vi "ExecLog_AddLogEntry.vi"(2 "Msg":string, 4 "EnableListDisplay":bool, 5 "Reset":bool, 6 "ReadLog":bool, 7 "FileRef":refnum<file>, 8 "error in":errorcluster, 9 "Force":bool, 10 "Code":i16=-1, 11 "Enable":bool) -> (0 "Log":string[][](array[string]), 1 "NewMsg":bool, 3 "ErrorOut":errorcluster)   [LabVIEW 2017]
doc: "Adds a log entry.\nFilters out duplicate messages and includes only the first and last. Duplicates can be either identified by identical text or by the same error code.\nCode is only ignored if zero."
uses:
  ExecLog_Type.ctl
panel:
  in  "LogType":T1
  out "call chain 2":string[](array[string])
  in  "Multicolumn Listbox":i32(listbox)
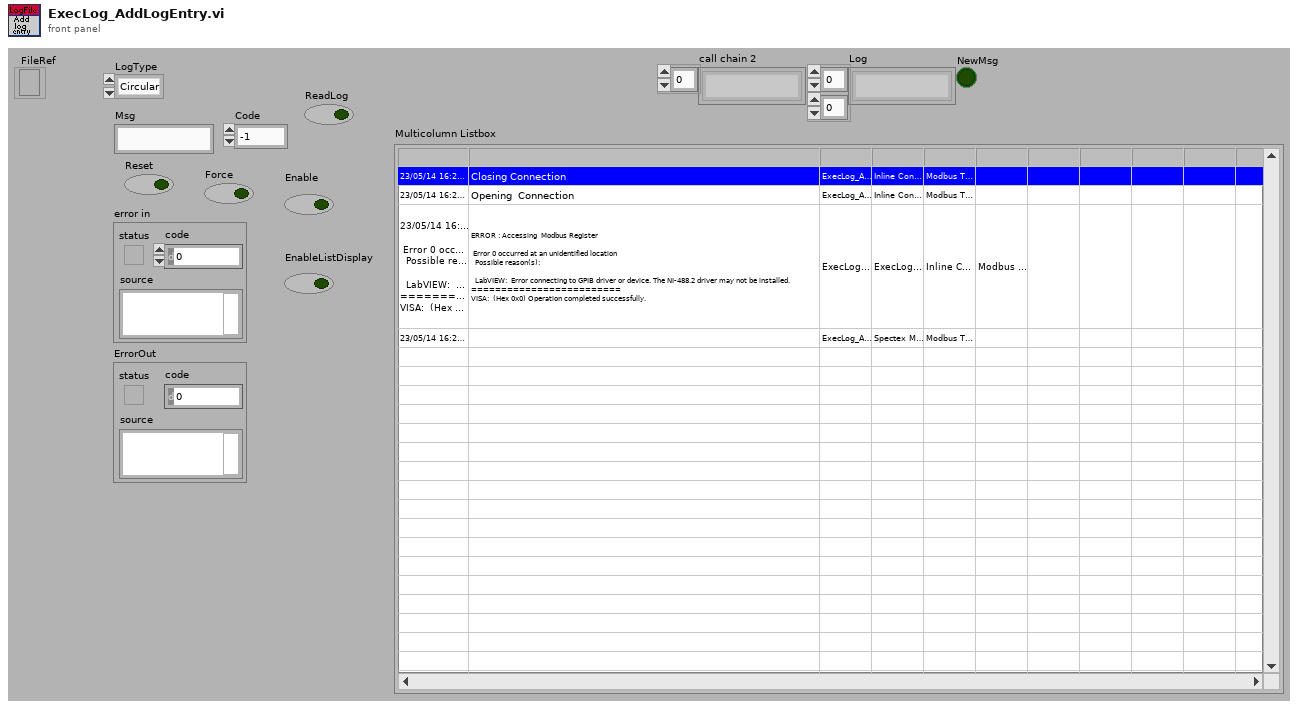
[diagram p1: front panel]
types:
  T1 = typedef "ExecLog_Type.ctl" = enum16{"Circular", "Daily"}
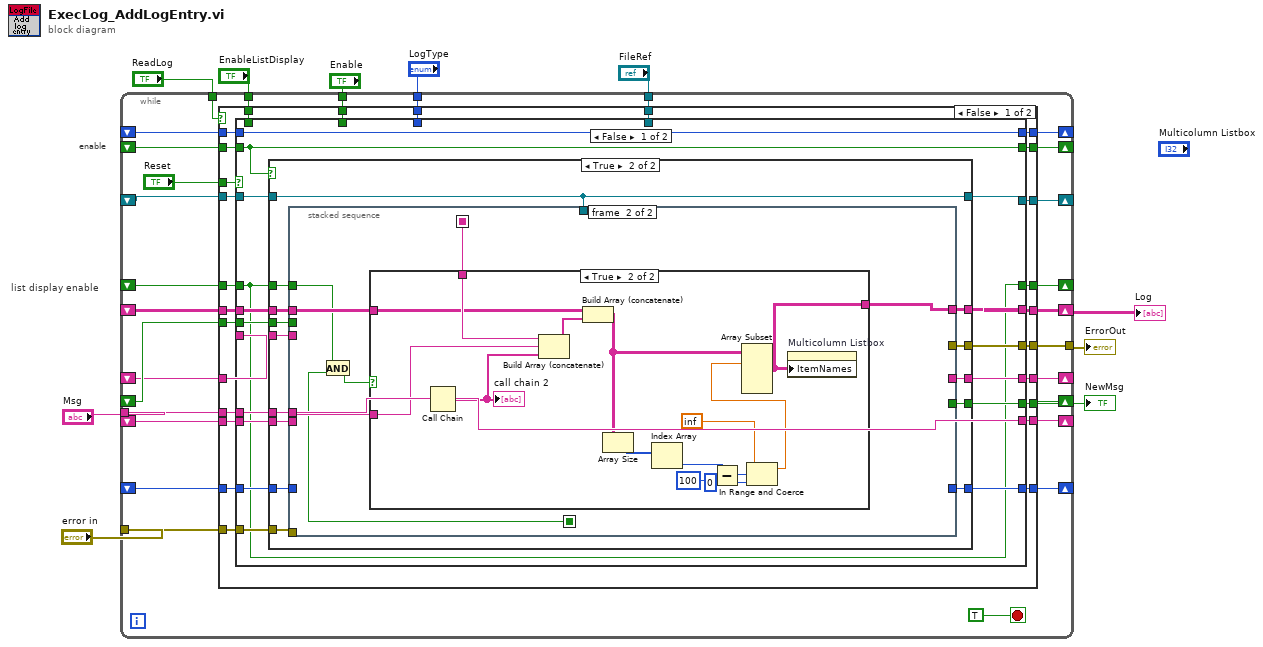
[diagram p0: block diagram]
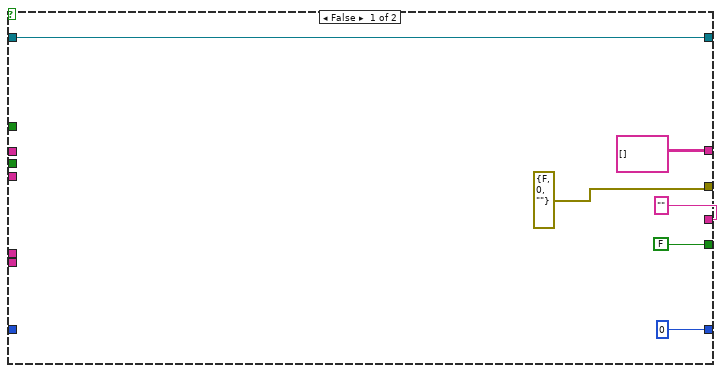
[diagram p2: hidden frame]
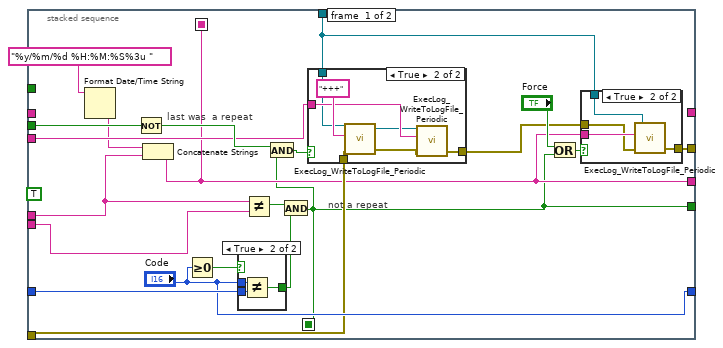
[diagram p3: hidden frame]
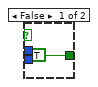
[diagram p4: hidden frame]
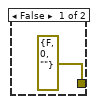
[diagram p6: hidden frame]
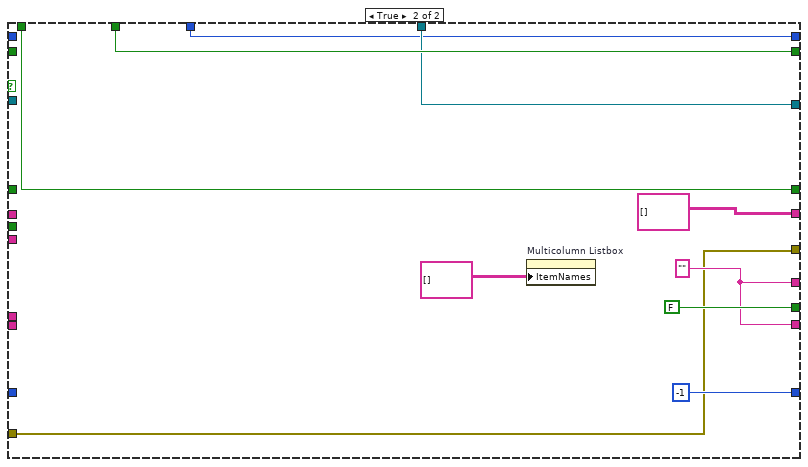
[diagram p8: hidden frame]
diagram:
  # "list display enable"
  # "enable"
  n1 = while {
    shift-right: [w30] -> _
    shift-left: _ -> [w37]
    tunnel: "Msg" -> [w38]
    shift-right: [w35] -> _
    shift-left: _ -> [w32]
    shift-right: [w33] -> w6
    shift-left: _ -> [w34]
    shift-right: [w28] -> _
    shift-left: _ -> [w29]
    tunnel: "error in" -> [w27]
    tunnel: [w26] -> w8
    shift-right: [w25] -> w7
    shift-left: _ -> [w24]
    shift-right: [w23] -> _
    shift-left: _ -> [w22]
    shift-right: [w20] -> _
    shift-left: _ -> [w18]
    tunnel: "Enable" -> [w21]
    tunnel: "EnableListDisplay" -> [w19]
    shift-right: [w17] -> _
    shift-left: _ -> [w15]
    tunnel: "FileRef" -> [w16]
    shift-right: [w14] -> _
    shift-left: _ -> [w12]
    tunnel: "LogType" -> [w13]
    tunnel: "ReadLog" -> [w11]
    stop <- TRUE stop-if-true
    n2 = case shown="False" w11 {
      tunnel: w38 -> [w64 _]
      tunnel: w37 -> [w63 w173]
      tunnel: [w62 w174] -> w35
      tunnel: w34 -> [w61 _]
      tunnel: [w60 _] -> w33
      tunnel: w32 -> [w59 w174]
      tunnel: "Reset" -> [w58 _]
      tunnel: [w57 w173] -> w30
      tunnel: w29 -> [w56 w172]
      tunnel: [w55 w172] -> w28
      tunnel: w27 -> [w54 _]
      tunnel: [w53 _] -> w26
      tunnel: [w52 w175] -> w25
      tunnel: w24 -> [w51 w175]
      tunnel: [w50 w178] -> w23
      tunnel: w22 -> [w49 w178]
      tunnel: w21 -> [w48 _]
      tunnel: [w47 w176] -> w20
      tunnel: w19 -> [w46 _]
      tunnel: w18 -> [w45 w176]
      tunnel: [w44 w177] -> w17
      tunnel: w16 -> [w43 _]
      tunnel: w15 -> [w42 w177]
      tunnel: [w41 w179] -> w14
      tunnel: w13 -> [w40 _]
      tunnel: w12 -> [w39 w179]
      frame False {
        n3 = case shown="False" w58 {
          tunnel: w64 -> [w77 _]
          tunnel: w63 -> [w81 _]
          tunnel: [w80 w170] -> w62
          tunnel: w61 -> [w79 _]
          tunnel: [w74 FALSE] -> w60
          tunnel: w59 -> [w78 _]
          tunnel: [w77 w170] -> w57
          tunnel: w56 -> [w76 _]
          tunnel: [w75 i16 -1 ("Code")] -> w55
          tunnel: w54 -> [w73 w168]
          tunnel: [w72 w168] -> w53
          tunnel: [w71 string[][] []] -> w52
          tunnel: w51 -> [w70 _]
          tunnel: [w69 w165] -> w50
          tunnel: w49 -> [w69 _]
          tunnel: w48 -> [_ w165]
          tunnel: [w68 w164] -> w47
          tunnel: w46 -> [_ w164]
          tunnel: w45 -> [w68 _]
          tunnel: [w66 w163] -> w44
          tunnel: w43 -> [_ w163]
          tunnel: w42 -> [w67 _]
          tunnel: [w65 w162] -> w41
          tunnel: w40 -> [_ w162]
          tunnel: w39 -> [w65 _]
          frame False {
            n4 = case shown="True" w69 {
              tunnel: w81 -> [_ w101]
              tunnel: ["" w100] -> w80
              tunnel: w79 -> [_ w99]
              tunnel: w78 -> [_ w98]
              tunnel: w77 -> [_ w97]
              tunnel: w76 -> [_ w96]
              tunnel: [i16 0 ("Code") w95] -> w75
              tunnel: [FALSE w94] -> w74
              tunnel: w73 -> [_ w93]
              tunnel: [errorcluster {"status"=FALSE, "code"=0, "source"=""} ("error out") w92] -> w72
              tunnel: [string[][] [] w91] -> w71
              tunnel: w70 -> [_ w90]
              tunnel: w68 -> [_ w89]
              tunnel: w67 -> [w82 w88]
              tunnel: [w82 w88] -> w66
              frame False {
              }
              frame True {
                n5 = stacked-sequence {
                  seq-local: [w106 _] -> [_ w146]
                  seq-local: [w105 _] -> [_ w142]
                  tunnel: w101 -> [w122 _]
                  tunnel: [w106 _] -> w100
                  tunnel: w99 -> [w121 _]
                  tunnel: w98 -> [w118 _]
                  tunnel: w97 -> [w117 w145]
                  tunnel: w96 -> [w116 _]
                  tunnel: ["Code" _] -> w95
                  tunnel: [w105 _] -> w94
                  tunnel: w93 -> [w108 _]
                  tunnel: [w107 _] -> w92
                  tunnel: [_ w144] -> w91
                  tunnel: w90 -> [_ w143]
                  tunnel: w89 -> [_ w141]
                  tunnel: w88 -> [w104 _]
                  frame #0 {
                    (unwired) TRUE ("want seconds? (F)")
                    # "last was  a repeat"
                    # "not a repeat"
                    n6 = Format Date/Time String(time format string (%c)="%y/%m/%d %H:%M:%S%3u ") -> (date/time string=w102:string)  [unwired: 2 in]
                    n7 = Not(x=w121) -> (.not. x?=w119:bool)
                    n8 = Concatenate Strings(w102, w117) -> (w106:string)
                    n9 = Greater Or Equal To 0?(x="Code") -> (x >= 0?=w112:bool)
                    n10 = case shown="True" w112 {
                      tunnel: w116 -> [_ w126]
                      tunnel: [TRUE w125] -> w114
                      tunnel: "Code" -> [_ w124]
                      frame False {
                      }
                      frame True {
                        n11 = Not Equal?(x=w124, y=w126) -> (x != y?=w125:bool)
                      }
                    }
                    n12 = Not Equal?(x=w117, y=w122) -> (x != y?=w115:bool)
                    n13 = And(x=w115, y=w114) -> (x .and. y?=w105:bool)
                    n14 = And(x=w119, y=w105) -> (x .and. y?=w120:bool)
                    n15 = case shown="True" w120 {
                      tunnel: w118 -> [_ w138]
                      tunnel: [errorcluster {"status"=FALSE, "code"=0, "source"=""} ("error out") w137] -> w109
                      tunnel: w108 -> [_ w135]
                      tunnel: w104 -> [_ w134]
                      frame False {
                      }
                      frame True {
                        n16 = call "ExecLog_WriteToLogFile_Periodic.vi"("error in"=w135, "string"="+++" ("character string"), "FileRef"=w134) -> ("error out"=w136:errorcluster, "FileRefOut"=w133:refnum<file>)  [unwired: 2 out]
                        n17 = call "ExecLog_WriteToLogFile_Periodic.vi"("error in"=w136, "string"=w138, "FileRef"=w133) -> ("error out"=w137:errorcluster)  [unwired: 3 out]
                      }
                    }
                    n18 = Or(x="Force", y=w105) -> (x .or. y?=w110:bool)
                    n19 = case shown="True" w110 {
                      tunnel: w106 -> [_ w131]
                      tunnel: w109 -> [w127 w129]
                      tunnel: [w127 w130] -> w107
                      tunnel: w104 -> [_ w128]
                      frame False {
                      }
                      frame True {
                        n20 = call "ExecLog_WriteToLogFile_Periodic.vi"("error in"=w129, "string"=w131, "FileRef"=w128) -> ("error out"=w130:errorcluster)  [unwired: 3 out]
                      }
                    }
                  }
                  frame #1 {
                    n21 = And(x=w141, y=w142) -> (x .and. y?=w140:bool)
                    n22 = case shown="True" w140 {
                      tunnel: w146 -> [_ w161]
                      tunnel: w145 -> [_ w160]
                      tunnel: [w147 w148] -> w144
                      tunnel: w143 -> [w147 w151]
                      frame False {
                      }
                      frame True {
                        n23 = Call Chain() -> (call chain=w159:string[])
                        "call chain 2" <- w159
                        n24 = Build Array (concatenate)(w161, w160, w159) -> (w158:string[])
                        n25 = Build Array (concatenate)(w151, w158) -> (w152:string[][])
                        n26 = Array Size(array=w152) -> (size(s)=w150:i32[])
                        n27 = Index Array(array=w150) -> (element=w149:i32)  [unwired: 1 in]
                        n28 = Subtract(x=w149, y=100) -> (x-y=w156:i32)
                        n29 = In Range and Coerce(upper limit=inf, x=w156, lower limit=0) -> (coerced(x)=w153:dbl)  [unwired: 1 out]
                        n30 = Array Subset(array=w152, index (row)=w153) -> (w148:string[][])  [unwired: 3 in]
                        n31 = property on="Multicolumn Listbox" class="MCListbox (strict)"("ItemNames"=w148) -> ()  [unwired: 2 in, 2 out]
                      }
                    }
                  }
                }
              }
            }
          }
          frame True {
            w170 = ""
            n32 = property on="Multicolumn Listbox" class="MCListbox (strict)"("ItemNames"=string[][] [] ("Item Names")) -> ()  [unwired: 2 in, 2 out]
          }
        }
      }
      frame True {
      }
    }
  }
  "ErrorOut" <- w8
  "Log" <- w7
  "NewMsg" <- w6
